vi "libssh2_init.vi"(8 "error in (no error)":errorcluster) -> (0 "error out":errorcluster, 3 "return value":i32)   [LabVIEW 2013, in "libssh2.lvlib"]
uses:
  libssh2.lvlib
  libssh2.dll
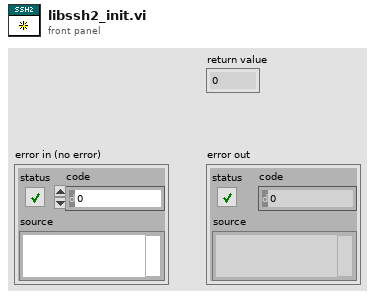
[diagram p1: front panel]
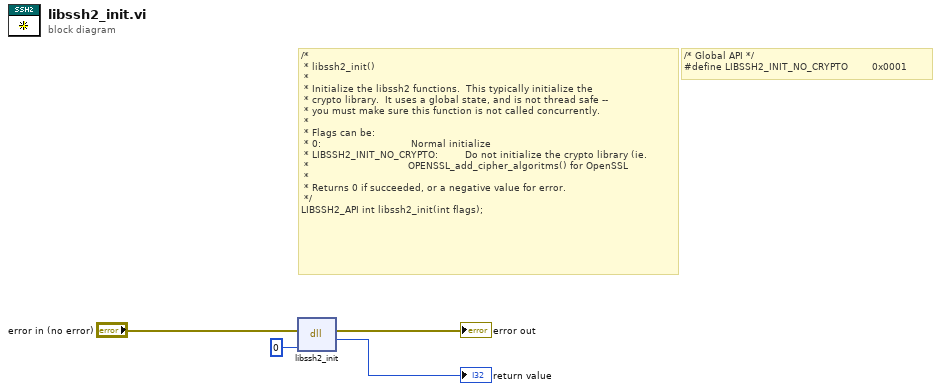
[diagram p0: block diagram]
diagram:
  # "/* Global API */\n#define LIBSSH2_INIT_NO_CRYPTO        0x0001"
  # "/*\n * libssh2_init()\n *\n * Initialize the libssh2 functions.  This typically initialize the\n * crypto library.  It uses a global state, and is not thread safe --\n * you must make sure this function is not called concurrently.\n *\n * Flags can be:\n * 0:                              Normal initialize\n * LIBSSH2_INIT_NO_CRYPTO:         Do not initialize the crypto library (ie.\n *                                 OPENSSL_add_cipher_algoritms() for OpenSSL\n *\n * Returns 0 if succeeded, or a negative value for error.\n */\nLIBSSH2_API int libssh2_init(int flags);"
  n1 = dll-call lib="C:/Users/pasca/OneDrive/LabVIEW/libssh2/libssh2**.*" fn="libssh2_init"(error in="error in (no error)", "flags"=0) -> (error out=→"error out":errorcluster, "return value"=→"return value":i32)  [unwired: 3 in, 1 out]
